vi "Write PORT.vi"(8 "error in (no error)":errorcluster, 10 "PORT":u16, 11 "Host Adapter in":refnum<class "Host Adapter.lvclass">) -> (0 "error out":errorcluster, 3 "Host Adapter out":refnum<class "Host Adapter.lvclass">)   [LabVIEW 2016, in "Host Adapter.lvlib" / "Host Adapter.lvclass"]
uses:
  Host Adapter.lvclass
  Host Adapter.lvclass/Host Adapter.ctl
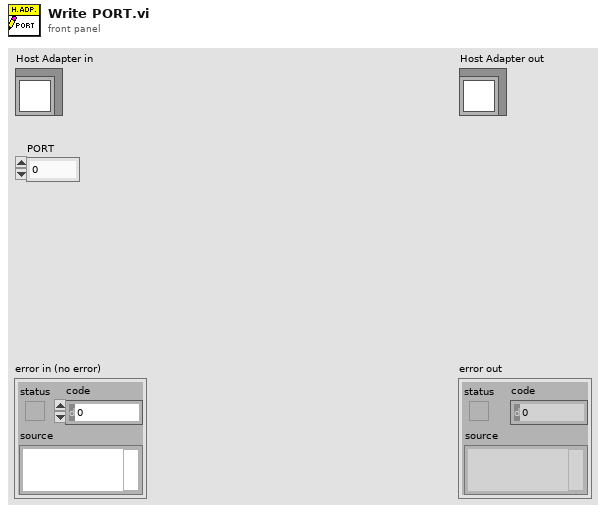
[diagram p1: front panel]
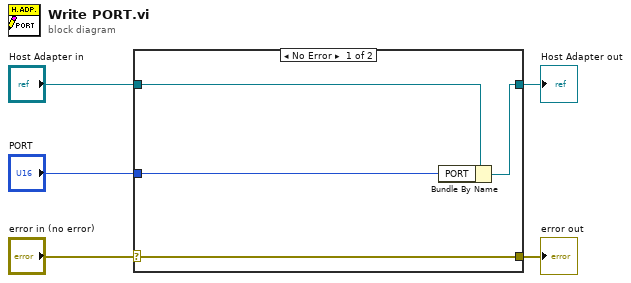
[diagram p0: block diagram]
diagram:
  n1 = case shown="No Error" "error in (no error)" {
    selector: "error in (no error)" -> [w9 w10]
    tunnel: [w9 w10] -> w4
    tunnel: [w7 w11] -> w2
    tunnel: "Host Adapter in" -> [w8 w11]
    tunnel: "PORT" -> [w6 _]
    frame No Error {
      n2 = Bundle By Name(cluster=w8, "PORT"=w6) -> (w7:refnum<class "Host Adapter.lvclass">)
    }
    frame Error {
    }
  }
  "error out" <- w4
  "Host Adapter out" <- w2
